vi "get runtime class name.vi"(8 "error in":errorcluster, 11 "fixed module parent implementation configuration in":refnum<class "fixed channel configuration.lvclass">) -> (0 "error out":errorcluster, 2 "class name":string, 3 "fixed module parent implementation configuration out":refnum<class "fixed channel configuration.lvclass">)   [LabVIEW 2013, in "fixed channel configuration.lvclass"]
doc: "Provides an interface for determining the module runtime class associated with this module configuration. This class name can then be used to dynamically load or locate the runtime class for initialization purposes."
uses:
  fixed channel configuration.lvclass
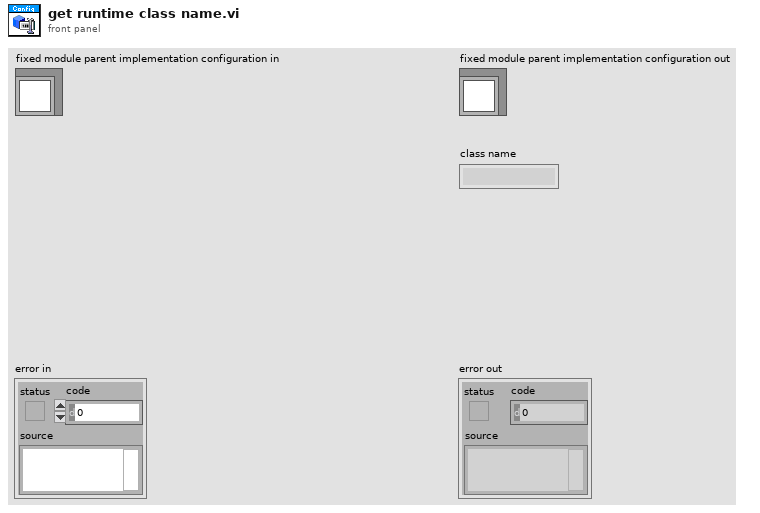
[diagram p1: front panel]
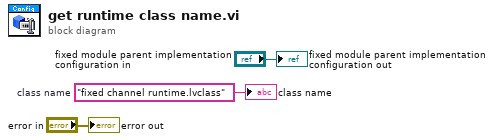
[diagram p0: block diagram]
diagram:
  w1 = "fixed channel runtime.lvclass"  # class name
  "error out" <- "error in"
  "fixed module parent implementation configuration out" <- "fixed module parent implementation configuration in"
  "class name" <- w1
